vi "CreateEvents.vi"(8 "error in (no error)":errorcluster, 11 "JQMHCore in":refnum<class "TesterModule.lvclass">) -> (0 "error out":errorcluster, 3 "JQMHCore out":refnum<class "TesterModule.lvclass">)   [LabVIEW 2024, in "TesterModule.lvclass"]
uses:
  TesterModule.lvclass
  TesterModule.lvclass/TesterModule.ctl
  JQMHCore/Module/JQMHModule.lvclass
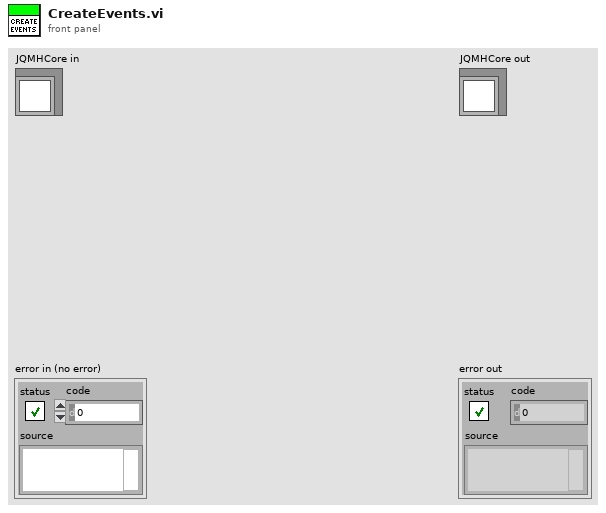
[diagram p1: front panel]
types:
  T1 = typedef "TesterModule.lvclass/Broadcast Events--cluster.ctl" = cluster{"Stopped":refnum<user-event>}
  T2 = typedef "TesterModule.lvclass/Request Events--cluster.ctl" = cluster{"Stopped":refnum<user-event>}
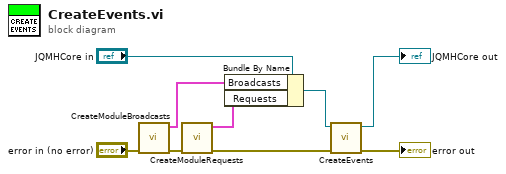
[diagram p0: block diagram]
diagram:
  n1 = call "CreateModuleBroadcasts.vi"("error in (no error)"="error in (no error)") -> ("error out"=w2:errorcluster, "Broadcasts"=w4:T1)  [unwired: 9 in]
  n2 = call "CreateModuleRequests.vi"("error in (no error)"=w2) -> ("error out"=w1:errorcluster, "Requests"=w3:T2)  [unwired: 9 in]
  n3 = Bundle By Name(cluster="JQMHCore in", "Broadcasts"=w4, "Requests"=w3) -> (w6:refnum<class "TesterModule.lvclass">)
  n4 = call-parent "CreateEvents.vi"("error in (no error)"=w1, "JQMHCore in"=w6) -> ("error out"=→"error out":errorcluster, "JQMHCore out"=→"JQMHCore out":refnum<class "TesterModule.lvclass">)  [unwired: 8 in]
